vi "Kickforce.vi"(8 "AI Parameters":T1={"GotoKick"={"Dist do cone a frente"=150.0, "attacker farback"=1500.0, "Perto"=300.0, "min dist to kick"=150.0, "kick eps"=0.05, "Time to transition"=0.0}, "Attacker"={"CC chute"=0.09, "CC passe"=0.045, "Kick Force"=100.0, "ball-robot Kick"=200.0, "ball-robot Pass"=0.3, "drible\nAttk"=FALSE}, "Defender"={"D max"=1700.0, "Vel p/ robô av"=1000.0, "Kick Force"=100.0, "D atk-def"=0.0, "D farback"=0.0, "drible\ndef"=FALSE, "drible\ngoalie"=FALSE}, "Timeout"={"Field/v in x"=6.0, "Dist Robots"=300, "Dist up in y"=300}, "Pose Striker"={"dist"=200.0, "Numeric"=-4.0, "dist 2"=200.0, "drible\nstriker"=FALSE}, "Dist Stop"=300.0, "D ball out"=200, "D central gap "=150.0, "T pass"=0.0, "Force ++"=0.0, "range kick"=0.0, "Chute alto"=TRUE, "Marcador novo"=TRUE, "drible"=FALSE, "D drible"=300.0, "Versão Striker"=enum."Auto", "Defesa"=enum."ManMark", "Marcador"=enum."Marcar Segundo mais perigoso", "Receptor passe"=enum."Auto", "Área"=enum."Quadrada", "Decisão\nsimples?"=FALSE} {"D drible" format="%#_13g"; "D central gap" format="%#_13g"; "Dist Stop" format="%#_13g"; "Pose Striker"."Numeric" format="%#_13g"; "Defender"."Kick Force" format="%#_13g"; "Defender"."Vel p/ robô av" format="%#_13g"; "Attacker"."ball-robot Kick" format="%#_13g"; "Attacker"."Kick Force" format="%#_13g"; "Attacker"."CC passe" format="%#_13g"; "Attacker"."CC chute" format="%#_13g"; "GotoKick"."kick eps" format="%#_13g"; "GotoKick"."min dist to kick" format="%#_13g"; "GotoKick"."Perto" format="%#_13g"; "GotoKick"."attacker farback" format="%#_13g"; "GotoKick"."Dist do cone a frente" format="%#_13g"}, 10 "Distância ao\nalvo do chute":dbl=1.23 format="%#_13g") -> (1 "Tempo até  bola\nchegar ao alvo":dbl, 2 "Força do chute":dbl)   [LabVIEW 2018]
uses:
  AI Parameters.ctl
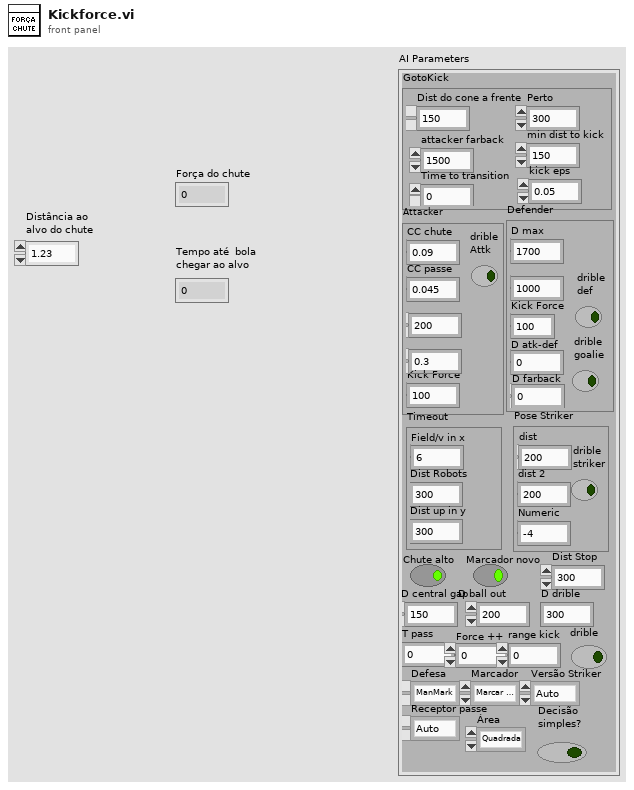
[diagram p1: front panel]
types:
  T1 = typedef "AI Parameters.ctl" = cluster{"GotoKick":cluster{"Dist do cone a frente":dbl, "attacker farback":dbl, "Perto":dbl, "min dist to kick":dbl, "kick eps":dbl, "Time to transition":dbl}, "Attacker":cluster{"CC chute":dbl, "CC passe":dbl, "Kick Force":dbl, "ball-robot Kick":dbl, "ball-robot Pass":dbl, "drible\nAttk":bool}, "Defender":cluster{"D max":dbl, "Vel p/ robô av":dbl, "Kick Force":dbl, "D atk-def":dbl, "D farback":dbl, "drible\ndef":bool, "drible\ngoalie":bool}, "Timeout":cluster{"Field/v in x":dbl, "Dist Robots":u32, "Dist up in y":u32}, "Pose Striker":cluster{"dist":dbl, "Numeric":dbl, "dist 2":dbl, "drible\nstriker":bool}, "Dist Stop":dbl, "D ball out":i32, "D central gap ":dbl, "T pass":dbl, "Force ++":dbl, "range kick":dbl, "Chute alto":bool, "Marcador novo":bool, "drible":bool, "D drible":dbl, "Versão Striker":enum16{"Auto", "3", "2", "1"}, "Defesa":enum16{"ManMark", "Barreira"}, "Marcador":enum16{"Marcar Segundo mais perigoso", "Marcar o mais perigoso"}, "Receptor passe":enum16{"Auto", "2nd Striker", "Striker"}, "Área":enum16{"Quadrada", "Circular"}, "Decisão\nsimples?":bool}
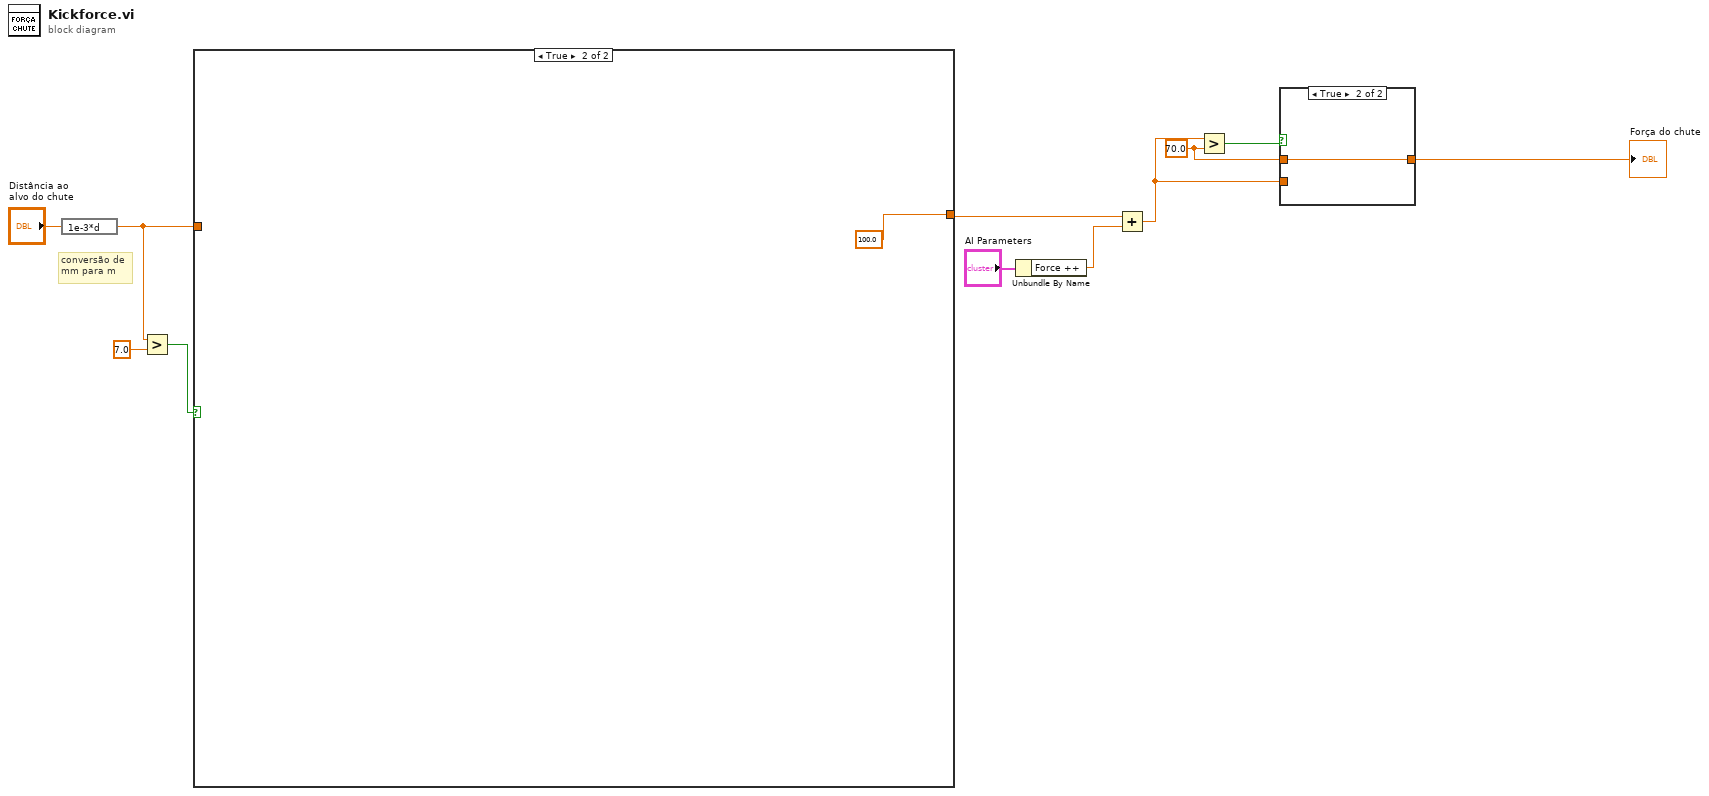
[diagram p0: block diagram]
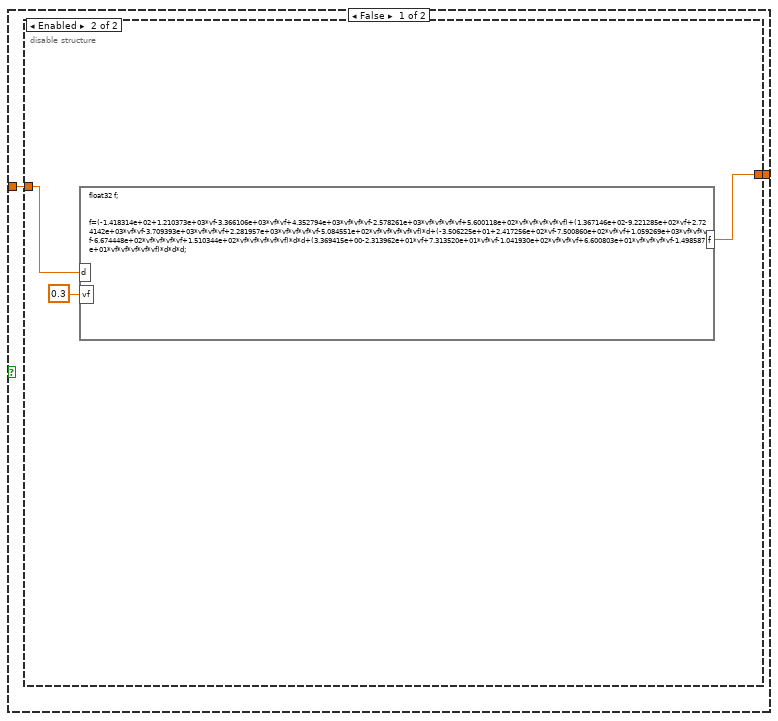
[diagram p3: hidden frame]
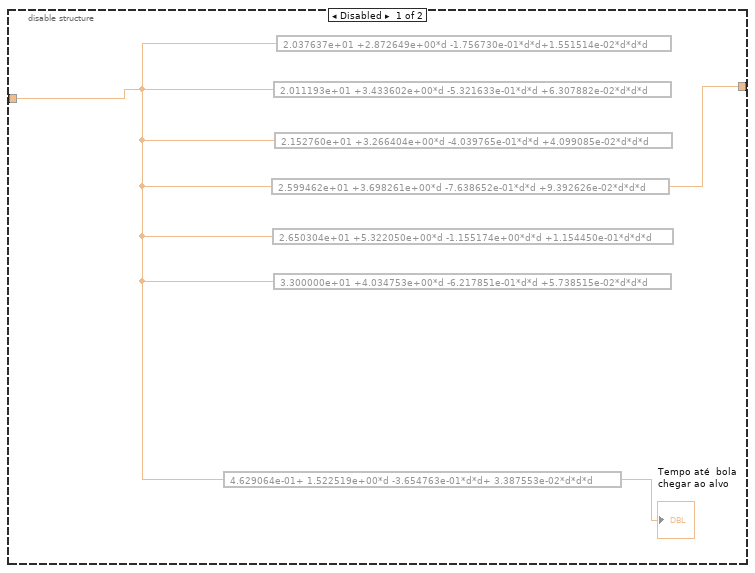
[diagram p4: hidden frame]
diagram:
  w1 = 70.0 ("y")
  # "conversão de\nmm para m"
  n1 = expression code="1e-3*d"("Distância ao\nalvo do chute") -> (w9:dbl)
  n2 = Greater?(x=w9, y=7.0) -> (0:w7:bool)
  n3 = case shown="True" w7 {
    tunnel: w9 -> [w13 _]
    tunnel: [w12 100.0] -> w10
    frame False {
      n4 = disable-structure shown="Enabled" {
        disable-tunnel: w13 -> [w16 w19]
        disable-tunnel: [w14 w18] -> w12
        frame Disabled {
          n5 = expression code="4.629064e-01+ 1.522519e+00*d -3.654763e-01*d*d+ 3.387553e-02*d*d*d"(w16) -> (→"Tempo até  bola\nchegar ao alvo":dbl)
          n6 = expression code="2.599462e+01 +3.698261e+00*d -7.638652e-01*d*d +9.392626e-02*d*d*d"(w16) -> (w14:dbl)
          n7 = expression code="2.650304e+01 +5.322050e+00*d -1.155174e+00*d*d +1.154450e-01*d*d*d"(w16) -> ()  [unwired: 1 out]
          n8 = expression code="2.011193e+01 +3.433602e+00*d -5.321633e-01*d*d +6.307882e-02*d*d*d"(w16) -> ()  [unwired: 1 out]
          n9 = expression code="3.300000e+01 +4.034753e+00*d -6.217851e-01*d*d +5.738515e-02*d*d*d"(w16) -> ()  [unwired: 1 out]
          n10 = expression code="2.152760e+01 +3.266404e+00*d -4.039765e-01*d*d +4.099085e-02*d*d*d"(w16) -> ()  [unwired: 1 out]
          n11 = expression code="2.037637e+01 +2.872649e+00*d -1.756730e-01*d*d+1.551514e-02*d*d*d"(w16) -> ()  [unwired: 1 out]
        }
        frame Enabled {
          n12 = formula code="float32 f;\n\n\nf=(-1.418314e+02+1.210373e+03*vf-3.366106e+03*vf*vf+4.352794e+03*vf*vf*vf-2.578261e+03*vf*vf*vf*vf+5.600118e+02*vf*vf*vf*vf*vf)+(1.367146e+02-9.221285e+02*vf+2.724142e+03*vf*vf-3.709393e+03*vf*vf*vf+2.281957e+03*vf*vf*vf*vf-5.084551e+02*vf*vf*vf*vf*vf)*d+(-3.506225e+01+2.417256e+02*vf-7.500860e+02*vf*vf+1.059269e+03*vf*vf*vf-6.674448e+02*vf*vf*vf*vf+1.510344e+02*vf*vf*vf*vf*vf)*d*d+(3.369415e+00-2.313962e+01*vf+7.313520e+01*vf*vf-1.041930e+02*vf*vf*vf+6.600803e+01*vf*vf*vf*vf-1.498587e+01*vf*vf*vf*vf*vf)*d*d*d;"("d"=w19, "vf"=0.3 ("input variable")) -> ("f"=w18:sgl)
        }
      }
    }
    frame True {
    }
  }
  n13 = Unbundle By Name("AI Parameters") -> ("Force ++"=w5:dbl)
  n14 = Add(x=w10, y=w5) -> (x+y=w2:dbl)
  n15 = Greater?(x=w2, y=w1) -> (0:w4:bool)
  n16 = case shown="True" w4 {
    tunnel: [w21 w22] -> w3
    tunnel: w2 -> [w21 _]
    tunnel: w1 -> [_ w22]
    frame False {
    }
    frame True {
    }
  }
  "Força do chute" <- w3
